vi "intake Controller.vi"(8 "error in":errorcluster) -> ()   [LabVIEW 2015]
doc: "This VI executes continuously carrying out the current operation and responding to updates or new operations. It will often contain the timing or control code that is difficult to place directly in TeleOp. This VI generally opens all sensors and motors and isolates the rest of the robot code from knowing how the operations are carried out."
uses:
  intake Setpoints.ctl
  intake Operations.ctl
  <vilib>/Rock Robotics/WPI/SafetyOutput/WPI_SafetyOutputConfigMenu.ctl
  <vilib>/Rock Robotics/SystemInterfaces/DIO/FPGA_DIOChannel.ctl
  <vilib>/Rock Robotics/WPI/Solenoid/WPI_SolenoidChannel.ctl
  <vilib>/Rock Robotics/WPI/Solenoid/WPI_SolenoidValue.ctl
  <vilib>/Rock Robotics/WPI/MotorControl/WPI_MotorControlOpenCANTalonSRX.vi
  <vilib>/Rock Robotics/WPI/Solenoid/WPI_SolenoidOpenDouble.vi
  <vilib>/Rock Robotics/WPI/Solenoid/WPI_SolenoidSetEnum.vi
  <vilib>/Rock Robotics/Network Tables/NT Write Boolean.vi
panel:
  out "Current\nCmd":string
  # "Tip: It may be helpful to observe inputs and sensor values.\nYou may also want to display tuning or debugging controls."
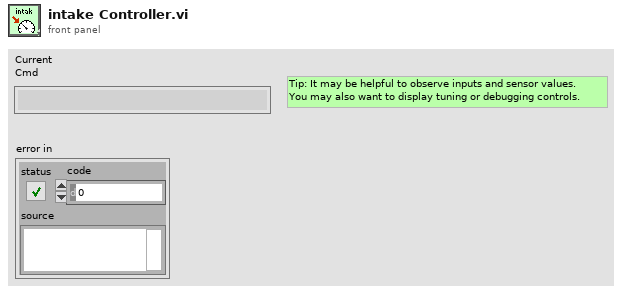
[diagram p1: front panel]
types:
  T1 = typedef "WPI_SolenoidChannel.ctl" = enum8{"Solenoid 0", "Solenoid 1", "Solenoid 2", "Solenoid 3", "Solenoid 4", "Solenoid 5", "Solenoid 6", "Solenoid 7", "Invalid"}
  T2 = typedef "FPGA_DIOChannel.ctl" = enum8{"DIO 0", "DIO 1", "DIO 2", "DIO 3", "DIO 4", "DIO 5", "DIO 6", "DIO 7", "DIO 8", "DIO 9", "DIO MXP 0", "DIO MXP 1", "DIO MXP 2", "DIO MXP 3", "DIO MXP 4", "DIO MXP 5", "DIO MXP 6", "DIO MXP 7", "DIO MXP 8", "DIO MXP 9", "DIO MXP 10", "DIO MXP 11", "DIO MXP 12", "DIO MXP 13", "DIO MXP 14", "DIO MXP 15", "Invalid"}
  T3 = typedef "WPI_SafetyOutputConfigMenu.ctl" = enum16{"Enable", "Disable"}
  T4 = typedef "intake Setpoints.ctl" = cluster{"Operation":T5, "Setpoint":dbl, "Duration":dbl, "up/down":dbl, "E-STOP":dbl, "Low goal?":dbl}
  T5 = typedef "intake Operations.ctl" = enum16{"Reserve", "Read Current", "move down/up", "Low Goal", "Shoot with intake", "pick up"}
  T6 = typedef "WPI_MotorControlDeviceRef.ctl" = cluster{"DeviceStatus":errorcluster, "Type":T7, "PWM":cluster{"PWM Channel":T8, "DeadBand":T9}, "CAN":cluster{"Device Number":u8, "Control Mode":T10, "Semaphore":T11, "Max Vout":dbl, "TalonSRX Control Mode":T12}, "Invert":bool}
  T7 = typedef "WPI_MotorControlType.ctl" = enum16{"PWM", "CAN", "CANTalonSRX"}
  T8 = typedef "FPGA_DIOPWMChannel.ctl" = enum8{"PWM 0", "PWM 1", "PWM 2", "PWM 3", "PWM 4", "PWM 5", "PWM 6", "PWM 7", "PWM 8", "PWM 9", "PWM MXP 0", "PWM MXP 1", "PWM MXP 2", "PWM MXP 3", "PWM MXP 4", "PWM MXP 5", "PWM MXP 6", "PWM MXP 7", "PWM MXP 8", "PWM MXP 9", "Invalid"}
  T9 = typedef "WPI_PWMDeadband.ctl" = cluster{"Name":string, "maxPositivePwm":i32, "minPositivePwm":i32, "centerPwm":i32, "maxNegativePwm":i32, "minNegativePwm":i32, "angularRange":u16}
  T10 = typedef "WPI_CANJaguar_ControlMode.ctl" = enum8{"Percent VBus", "Current", "Speed", "Position", "Voltage"}
  T11 = typedef "Semaphore RefNum" = refnum<k1>
  T12 = typedef "WPI_CANTalonSRX_APIControlMode.ctl" = enum8{"Percent VBus", "Speed", "Position", "Slave", "Unchanged / Invalid", "Voltage Compensation", "Current", "Motion Profile"}
  T13 = typedef "WPI_DigitalInputDevRef.ctl" = cluster{"DevStatus":errorcluster, "DIO Channel":T2}
  T14 = typedef "WPI_SolenoidDevRef.ctl" = cluster{"DevStatus":errorcluster, "Pneumatics Control Module":u8, "Forward Solenoid Channel":T1, "Reverse Solenoid Channel":T1}
  T15 = typedef "Command Status Info.ctl" = cluster{"Name":string, "Status":T16, "notifier out":T17}
  T16 = typedef "Completion Status.ctl" = enum16{"Successful", "Aborted", "Incomplete"}
  T17 = typedef "Completion Notifier.ctl" = refnum<notifier>
  T18 = cluster{"Default Command":T4, "Command Timing":cluster{"Start Time (ms)":u32, "Iterations":i32}, "Command Arguments":cluster{"Command Info":T15, "Description":string, "Default Command":T4, "notifier out":refnum<notifier>, "Subsystem Name":string}}
  T19 = typedef "WPI_SolenoidValue.ctl" = enum16{"Off", "On", "Forward", "Reverse"}
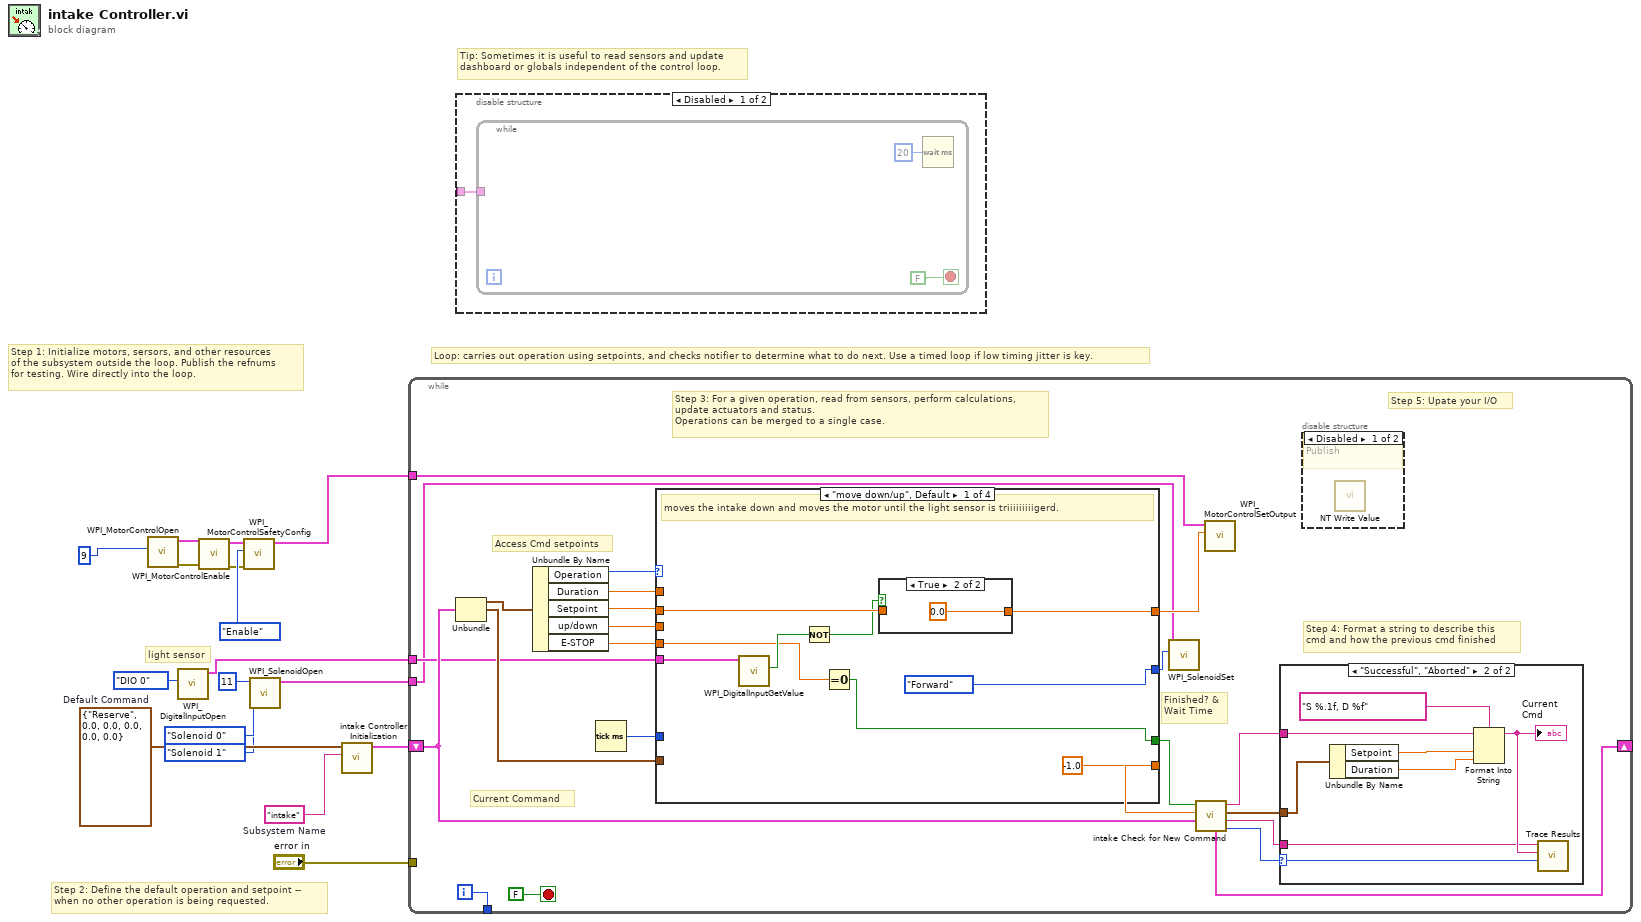
[diagram p0: block diagram]
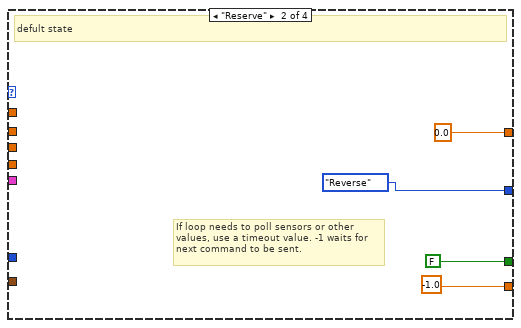
[diagram p6: hidden frame]
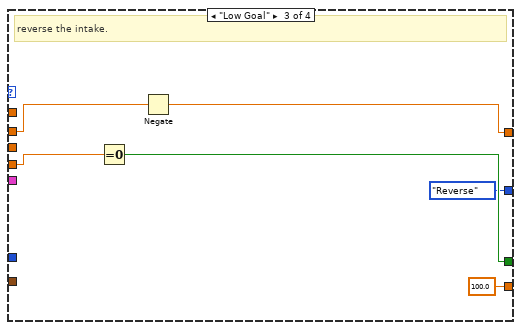
[diagram p7: hidden frame]
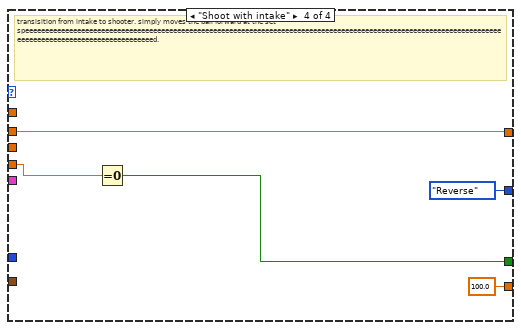
[diagram p8: hidden frame]
diagram:
  w14 = T4 {"Operation"=enum."Reserve", "Setpoint"=0.0, "Duration"=0.0, "up/down"=0.0, "E-STOP"=0.0, "Low goal?"=0.0}  # Default Command
  w15 = "intake"  # Subsystem Name
  # "light sensor"
  # "Tip: Sometimes it is useful to read sensors and update\ndashboard or globals independent of the control loop."
  # "Step 2: Define the default operation and setpoint --\nwhen no other operation is being requested."
  # "Step 1: Initialize motors, sersors, and other resources\nof the subsystem outside the loop. Publish the refnums\nfor testing. Wire directly into the loop."
  # "Loop: carries out operation using setpoints, and checks notifier to determine what to do next. Use a timed loop if low timing jitter is key."
  n1 = call-poly <vilib>:"WPI_MotorControlOpen.vi"("Device Number"=u8 9) -> ("error out"=w6:errorcluster, "MotorControlDeviceRef"=w13:T6)  [unwired: 9 in]
  n2 = call <vilib>:"WPI_DigitalInputOpen.vi"("DIO Channel"=FPGA_DIOChannel."DIO 0") -> ("DigitalInputDevRef"=w8:T13)  [unwired: 9 in, 1 out]
  n3 = call <vilib>:"WPI_MotorControlEnable.vi"("error in (no error)"=w6, "CAN MotorDevRef"=w13) -> ("error out"=w5:errorcluster, "CAN MotorDevRef"=w12:T6)  [unwired: 8 in]
  n4 = call <vilib>:"WPI_MotorControlSafetyConfig.vi"("error in (no error)"=w5, "mode"=WPI_SafetyOutputConfigMenu."Enable", "MotorControlDevRef"=w12) -> ("MotorControlDevRef"=w10:T6)  [unwired: 7 in, 1 out]
  n5 = call-poly <vilib>:"WPI_SolenoidOpen.vi"("Reverse Solenoid Channel"=WPI_SolenoidChannel."Solenoid 1", "Forward Solenoid Channel"=WPI_SolenoidChannel."Solenoid 0", "Pneumatics Control Module (0)"=u8 11) -> ("SolenoidDevRef"=w1:T14)  [unwired: 7 in, 1 out]
  n6 = call "intake Controller Initialization.vi"("Subsystem Name"=w15, "Default Command"=w14) -> ("Command Info"=w16:T18)  [unwired: 9 in]
  n7 = while {
    shift-right: [w32] -> _
    shift-left: w16 -> [w33]
    tunnel: [w39] -> _
    tunnel: "error in" -> [_]
    tunnel: w10 -> [w22]
    tunnel: w8 -> [w25]
    tunnel: w1 -> [w18]
    i -> [w39]
    stop <- FALSE stop-if-true
    # "Step 5: Upate your I/O"
    # "Step 4: Format a string to describe this\ncmd and how the previous cmd finished"
    # "Current Command"
    # "Access Cmd setpoints"
    # "Finished? &\nWait Time"
    # "Step 3: For a given operation, read from sensors, perform calculations,\nupdate actuators and status.\nOperations can be merged to a single case."
    n8 = Unbundle(w33) -> ("Default Command"=w38:T4, "Command Timing"=w34:cluster{"Start Time (ms)":u32, "Iterations":i32})  [unwired: 1 out]
    n9 = Unbundle By Name(w38) -> ("Operation"=w37:T5, "Duration"=w36:dbl, "Setpoint"=w23:dbl, "up/down"=w21:dbl, "E-STOP"=w20:dbl)
    n10 = Tick Count (ms)() -> (millisecond timer value=w35:u32)
    n11 = case shown="\"move down/up\", Default" w37 {
      tunnel: [-1.0 -1.0 100.0 100.0] -> w30
      tunnel: [w49 FALSE ("ignore previous (F)") w66 w71] -> w31
      tunnel: w34 -> [_ _ _ _]
      tunnel: w36 -> [_ _ _ _]
      tunnel: w35 -> [_ _ _ _]
      tunnel: w23 -> [w55 _ w69 w73]
      tunnel: w25 -> [w56 _ _ _]
      tunnel: [w54 0.0 ("Setpoint") w68 w73] -> w24
      tunnel: w21 -> [_ _ _ _]
      tunnel: w20 -> [w50 _ w67 w72]
      tunnel: [WPI_SolenoidValue."Forward" ("Value") WPI_SolenoidValue."Reverse" ("Value") WPI_SolenoidValue."Reverse" ("Value") WPI_SolenoidValue."Reverse" ("Value")] -> w19
      frame "move down/up", Default {
        # "moves the intake down and moves the motor until the light sensor is triiiiiiiiigerd."
        n12 = call <vilib>:"WPI_DigitalInputGetValue.vi"("DigitalInputDevRef"=w56) -> ("Value"=w53:bool)  [unwired: 8 in, 2 out]
        n13 = Not(x=w53) -> (.not. x?=w52:bool)
        n14 = Equal To 0?(x=w50) -> (x = 0?=w49:bool)
        n15 = case shown="True" w52 {
          tunnel: w55 -> [w58 _]
          tunnel: [w58 0.0] -> w54
          frame False {
          }
          frame True {
          }
        }
      }
      frame "Reserve" {
        # "If loop needs to poll sensors or other\nvalues, use a timeout value. -1 waits for\nnext command to be sent."
        # "defult state"
      }
      frame "Low Goal" {
        # "reverse the intake."
        n16 = Equal To 0?(x=w67) -> (x = 0?=w66:bool)
        n17 = Negate(x=w69) -> (-x=w68:dbl)
      }
      frame "Shoot with intake" {
        # "transisition from intake to shooter. simply moves the ball forward at the set speeeeeeeeeeeeeeeeeeeeeeeeeeeeeeeeeeeeeeeeeeeeeeeeeeeeeeeeeeeeeeeeeeeeeeeeeeeeeeeeeeeeeeeeeeeeeeeeeeeeeeeeeeeeeeeeeeeeeeeeeeeeeeeeeeeeeeeeeeeeeeeeeeeeeeeeed."
        n18 = Equal To 0?(x=w72) -> (x = 0?=w71:bool)
      }
    }
    n19 = call-poly <vilib>:"WPI_SolenoidSet.vi"("Value"=w19, "SolenoidDevRef"=w18) -> ()  [unwired: 8 in, 2 out]
    n20 = call "intake Check for New Command.vi"("Current Command"=w33, "Wait time (ms)"=w30, "Finished?"=w31) -> ("Completion"=w26:T16, "Subsystem Name"=w27:string, "Current Command"=w28:T4, "Initial Trace String"=w29:string, "NextCommand"=w32:T18)  [unwired: 4 in]
    n21 = call <vilib>:"WPI_MotorControlSetOutput.vi"("Output"=w24, "MotorControlDevRef"=w22) -> ()  [unwired: 7 in, 3 out]
    n22 = case shown="\"Successful\", \"Aborted\"" w26 {
      selector: w26 -> [_ w48]
      tunnel: w29 -> [_ w44]
      tunnel: w28 -> [_ w45]
      tunnel: w27 -> [_ w41]
      frame "Incomplete", Default {
        # "Continuing current command"
      }
      frame "Successful", "Aborted" {
        # "Report and setup for next command"
        n23 = Unbundle By Name(w45) -> ("Setpoint"=w47:dbl, "Duration"=w42:dbl)
        n24 = Format Into String(format string="S %.1f, D %f", initial string=w44, w47, w42) -> (resulting string=w43:string)  [unwired: 1 in, 1 out]
        "Current\nCmd" <- w43
        n25 = call <vilib>:"Trace Results.vi"("Status of previous command"=w48, "Description"=w43, "Subsystem"=w41) -> ()  [unwired: 9 in]
      }
    }
    n26 = disable-structure shown="Disabled" {
      frame Disabled {
        # "Publish"
        n27 = call-poly <vilib>:"NT Write Value.vi"() -> ()  [unwired: 11 in, 1 out]
      }
      frame Enabled {
      }
    }
  }
  n28 = disable-structure shown="Disabled" {
    disable-tunnel: _ -> [w75 _]
    frame Disabled {
      n29 = while {
        tunnel: w75 -> [_]
        stop <- FALSE stop-if-true
        n30 = Wait (ms)(milliseconds to wait=u32 20) -> ()  [unwired: 1 out]
      }
    }
    frame Enabled {
    }
  }
